vi "V70.vi"(7 "V70 VISA Source":string, 11 "V70 Write":string) -> (2 "OK?":bool, 3 "Response":string, 4 "error out":errorcluster)   [LabVIEW 2020, in "FBN_LATM.lvlib"]
uses:
  FBN_LATM.lvlib
  <vilib>/Instr/_visa.llb/VISA Configure Serial Port (Instr).vi
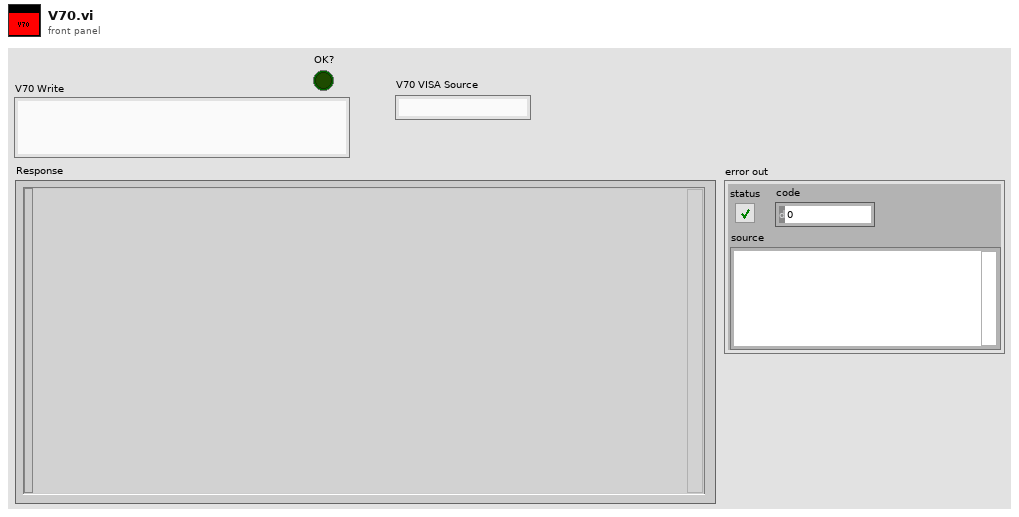
[diagram p1: front panel]
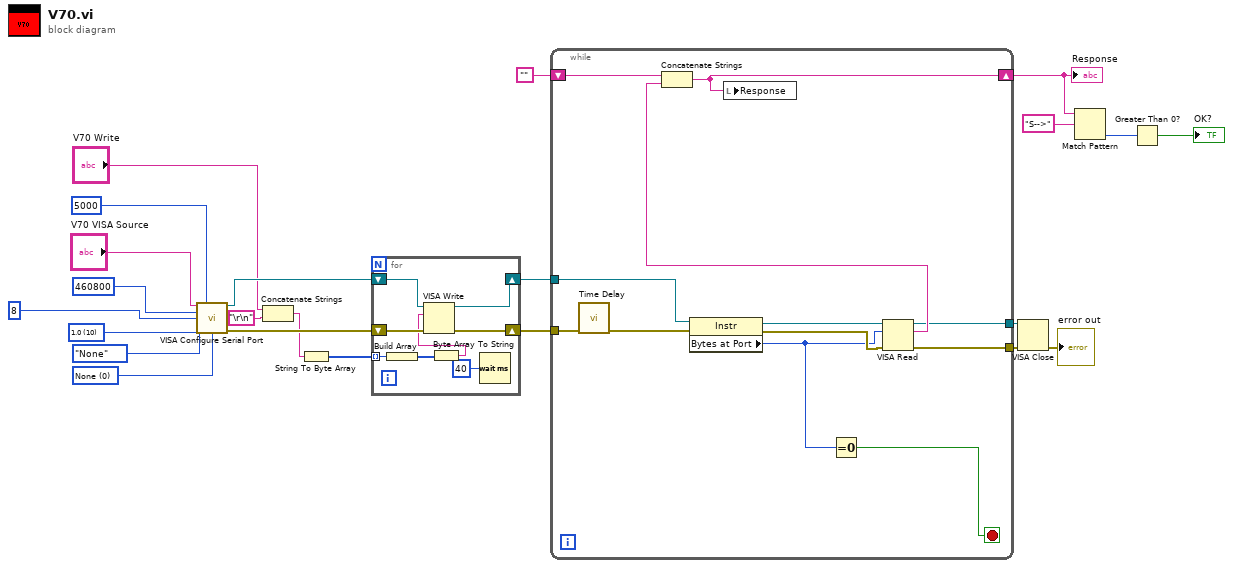
[diagram p0: block diagram]
diagram:
  w20 = u16 0 items=["None", "XON/XOFF", "RTS/CTS", "XON/XOFF & RTS/CTS", "DTR/DSR", "XON/XOFF & DTR/DSR"] ("flow control (0:none)")
  w21 = u16 10 items=["1.0"=10, "1.5"=15, "2.0"=20] ("stop bits (10: 1 bit)")
  n1 = call-poly "VISA Configure Serial Port"("VISA resource name"="V70 VISA Source", "timeout (10sec)"=u32 5000, "baud rate (9600)"=u32 460800, "data bits (8)"=u16 8, "parity (0:none)"=enum16{"None", "Odd", "Even", "Mark", "Space"}."None", "stop bits (10: 1 bit)"=w21, "flow control (0:none)"=w20) -> ("VISA resource name out"=w13:refnum<visa-resource-name>, "error out"=w14:errorcluster)  [unwired: 2 in, 5 out]
  n2 = Concatenate Strings("V70 Write", "\r\n") -> (w9:string)
  n3 = String To Byte Array(string=w9) -> (unsigned byte array=w8:u8[])
  n4 = for {
    shift-right: [w28] -> w12
    shift-left: w14 -> [w31]
    shift-right: [w29] -> w11
    shift-left: w13 -> [w30]
    tunnel: w8 -> [w27] mode=indexing
    n5 = Build Array(w27) -> (w26:u8[])
    n6 = Byte Array To String(unsigned byte array=w26) -> (string=w25:string)
    n7 = VISA Write(VISA resource name=w30, write buffer=w25, error in (no error)=w31) -> (VISA resource name out=w29:refnum<visa-resource-name>, error out=w28:errorcluster)  [unwired: 1 out]
    n8 = Wait (ms)(milliseconds to wait=u32 40) -> ()  [unwired: 1 out]
  }
  n9 = while {
    shift-right: [w41] -> w3
    shift-left: "" -> [w39]
    tunnel: [w37] -> w16
    tunnel: [w36] -> w15
    tunnel: w12 -> [w35]
    tunnel: w11 -> [w34]
    stop <- w32 stop-if-true
    n10 = call "Time Delay"("error in (no error)"=w35) -> ("error out"=w38:errorcluster)  [unwired: 10 in]
    n11 = property class="Instr"(reference=w34, error in=w38) -> (reference out=w43:refnum<visa-resource-name>, error out=w42:errorcluster, "Bytes at Port"=w33:u32)
    n12 = Equal To 0?(x=w33) -> (x = 0?=w32:bool)
    n13 = VISA Read(VISA resource name=w43, byte count=w33, error in (no error)=w42) -> (VISA resource name out=w36:refnum<visa-resource-name>, read buffer=w40:string, error out=w37:errorcluster)  [unwired: 1 out]
    n14 = Concatenate Strings(w39, w40) -> (w41:string)
    n15 = local write "Response"(w41) -> ()
  }
  "Response" <- w3
  n16 = VISA Close(VISA resource name=w15, error in (no error)=w16) -> (error out=→"error out":errorcluster)
  n17 = Match Pattern(string=w3, regular expression="S-->" ("replace string (\"\")")) -> (offset past match=w5:i32)  [unwired: 1 in, 3 out]
  n18 = Greater Than 0?(x=w5) -> (x > 0?=→"OK?":bool)
